vi "scan PZT_V(SubVI).vi"(0 "config":T1={"initialize"=enum."SR830", "6221"={"6221 Resource"="GPIB0::24::INSTR", "Delta status"=FALSE, "电流|RMS(A)"=0.0}, "SR830+6221"={"source"=0, "Current(A)"=0.0, "阻抗(Ohm)"=0.0, "SR830 1"=FALSE, "SR830 2"=FALSE, "SR830 3"=FALSE, "SR830 4"=FALSE, "VISA 1"="", "VISA 2"="", "VISA 3"="", "VISA 4"="", "Reserve 1"=0, "Reserve 2"=-1, "Reserve 3"=-1, "Reserve 4"=-1, "Sensitivity 1"=-1, "Sensitivity 2"=0, "Sensitivity 3"=-1, "Sensitivity 4"=-1, "量程入 1"=0, "量程入 2"=0, "量程入 3"=0, "量程入 4"=0}, "2400"={"2400"=FALSE, "VISA"="", "Output Level (0)"=1e-05, "Compliance  Level (0.1)"=10.0}, "ch"={"ch"=[], "current"=[], "change?"=[], "holding current\nwhen change ch?"=FALSE}, "Instrument"={"335 Resource"="GPIB0::24::INSTR", "Input (0:A)"=0, "Instrument Type"=enum."PPMS-Rotate", "quantum design"=refnum, "Heater Output (1:1)"=1, "semaphore"=refnum, "TCP master instance"=refnum, "335 Status"=refnum, "M24C Resource"="GPIB0::24::INSTR", "4G supply"="GPIB0::24::INSTR", "Temp Status 24C"=refnum, "Temp"=refnum, "9T信号"=refnum, "limit"={"Field limit"=0.0, "Field rate limit"=0.0, "Temp limit"=0.0, "Temp low limit"=0.0, "Temp rate limit "=0.0}, "4g supply status"=refnum, "vi路径"="", "325 Resource "="GPIB0::24::INSTR", "Input (0:A) 325"=0, "Input (1;B)"=1, "in-plane"="", "out-plane"="", "in-plane"=FALSE, "out-plane"=FALSE, "in plane 信号"=refnum, "pzt volt"=refnum, "Aborting"=refnum, "数据文件"=refnum, "warning"=refnum}, "2614B"={"2614B chA"=FALSE, "2614B chB"=FALSE, "VISA"=""}, "33522b"={"33522b resource name"="", "零电压"=0.0, "最大电压"=148.0, "间隔"=4.0, "最小电压"=-48.0, "PZT Scan?"=FALSE}, "gating type"=enum."2614(daul)"} {"Instrument"."Input (1;B)" items=["A", "B"]; "Instrument"."Input (0:A) 325" items=["A", "B"]; "Instrument"."Input (0:A)" items=["A", "B"]; "Instrument"."Heater Output (1:1)" items=["1"=1, "2"=2]; "SR830+6221"."Sensitivity 4" items=["Auto Gain"=-1, "2 nV/fA"=0, "5 nV/fA"=1, "10 nV/fA"=2, "20 nV/fA"=3, "50 nV/fA"=4, "100 nV/fA"=5, "200 nV/fA"=6, "500 nV/fA"=7, "1 uV/pA"=8, "2 uV/pA"=9, "5 uV/pA"=10, "10 uV/pA"=11, "20 uV/pA"=12, "50 uV/pA"=13, "100 uV/pA"=14, "200 uV/pA"=15, "500 uV/pA"=16, "1 mV/nA"=17, "2 mV/nA"=18, "5 mV/nA"=19, "10 mV/nA"=20, "20 mV/nA"=21, "50 mV/nA"=22, "100 mV/nA"=23, "200 mV/nA"=24, "500 mV/mA"=25, "1 V/uA"=26]; "SR830+6221"."Sensitivity 3" items=["Auto Gain"=-1, "2 nV/fA"=0, "5 nV/fA"=1, "10 nV/fA"=2, "20 nV/fA"=3, "50 nV/fA"=4, "100 nV/fA"=5, "200 nV/fA"=6, "500 nV/fA"=7, "1 uV/pA"=8, "2 uV/pA"=9, "5 uV/pA"=10, "10 uV/pA"=11, "20 uV/pA"=12, "50 uV/pA"=13, "100 uV/pA"=14, "200 uV/pA"=15, "500 uV/pA"=16, "1 mV/nA"=17, "2 mV/nA"=18, "5 mV/nA"=19, "10 mV/nA"=20, "20 mV/nA"=21, "50 mV/nA"=22, "100 mV/nA"=23, "200 mV/nA"=24, "500 mV/mA"=25, "1 V/uA"=26]; "SR830+6221"."Sensitivity 1" items=["Auto Gain"=-1, "2 nV/fA"=0, "5 nV/fA"=1, "10 nV/fA"=2, "20 nV/fA"=3, "50 nV/fA"=4, "100 nV/fA"=5, "200 nV/fA"=6, "500 nV/fA"=7, "1 uV/pA"=8, "2 uV/pA"=9, "5 uV/pA"=10, "10 uV/pA"=11, "20 uV/pA"=12, "50 uV/pA"=13, "100 uV/pA"=14, "200 uV/pA"=15, "500 uV/pA"=16, "1 mV/nA"=17, "2 mV/nA"=18, "5 mV/nA"=19, "10 mV/nA"=20, "20 mV/nA"=21, "50 mV/nA"=22, "100 mV/nA"=23, "200 mV/nA"=24, "500 mV/mA"=25, "1 V/uA"=26]; "SR830+6221"."Sensitivity 2" items=["Auto Gain"=-1, "2 nV/fA"=0, "5 nV/fA"=1, "10 nV/fA"=2, "20 nV/fA"=3, "50 nV/fA"=4, "100 nV/fA"=5, "200 nV/fA"=6, "500 nV/fA"=7, "1 uV/pA"=8, "2 uV/pA"=9, "5 uV/pA"=10, "10 uV/pA"=11, "20 uV/pA"=12, "50 uV/pA"=13, "100 uV/pA"=14, "200 uV/pA"=15, "500 uV/pA"=16, "1 mV/nA"=17, "2 mV/nA"=18, "5 mV/nA"=19, "10 mV/nA"=20, "20 mV/nA"=21, "50 mV/nA"=22, "100 mV/nA"=23, "200 mV/nA"=24, "500 mV/mA"=25, "1 V/uA"=26]; "SR830+6221"."Reserve 4" items=["Auto Gain"=-1, "2 nV/fA"=0, "5 nV/fA"=1, "10 nV/fA"=2, "20 nV/fA"=3, "50 nV/fA"=4, "100 nV/fA"=5, "200 nV/fA"=6, "500 nV/fA"=7, "1 uV/pA"=8, "2 uV/pA"=9, "5 uV/pA"=10, "10 uV/pA"=11, "20 uV/pA"=12, "50 uV/pA"=13, "100 uV/pA"=14, "200 uV/pA"=15, "500 uV/pA"=16, "1 mV/nA"=17, "2 mV/nA"=18, "5 mV/nA"=19, "10 mV/nA"=20, "20 mV/nA"=21, "50 mV/nA"=22, "100 mV/nA"=23, "200 mV/nA"=24, "500 mV/mA"=25, "1 V/uA"=26]; "SR830+6221"."Reserve 3" items=["Auto Reserve"=-1, "High Reserve"=0, "Normal"=1, "Low Noise"=2]; "SR830+6221"."Reserve 2" items=["Auto Reserve"=-1, "High Reserve"=0, "Normal"=1, "Low Noise"=2]; "SR830+6221"."Reserve 1" items=["Auto Reserve"=-1, "High Reserve"=0, "Normal"=1, "Low Noise"=2]; "SR830+6221"."source" items=["SR830 1", "SR830 2", "SR830 3", "SR830 4"]}, 12 "data":refnum<queue>) -> (4 "输出簇":T1={"initialize"=enum."SR830", "6221"={"6221 Resource"="GPIB0::24::INSTR", "Delta status"=FALSE, "电流|RMS(A)"=0.0}, "SR830+6221"={"source"=0, "Current(A)"=0.0, "阻抗(Ohm)"=0.0, "SR830 1"=FALSE, "SR830 2"=FALSE, "SR830 3"=FALSE, "SR830 4"=FALSE, "VISA 1"="", "VISA 2"="", "VISA 3"="", "VISA 4"="", "Reserve 1"=0, "Reserve 2"=-1, "Reserve 3"=-1, "Reserve 4"=-1, "Sensitivity 1"=-1, "Sensitivity 2"=0, "Sensitivity 3"=-1, "Sensitivity 4"=-1, "量程入 1"=0, "量程入 2"=0, "量程入 3"=0, "量程入 4"=0}, "2400"={"2400"=FALSE, "VISA"="", "Output Level (0)"=1e-05, "Compliance  Level (0.1)"=10.0}, "ch"={"ch"=[], "current"=[], "change?"=[], "holding current\nwhen change ch?"=FALSE}, "Instrument"={"335 Resource"="GPIB0::24::INSTR", "Input (0:A)"=0, "Instrument Type"=enum."PPMS-Rotate", "quantum design"=refnum, "Heater Output (1:1)"=1, "semaphore"=refnum, "TCP master instance"=refnum, "335 Status"=refnum, "M24C Resource"="GPIB0::24::INSTR", "4G supply"="GPIB0::24::INSTR", "Temp Status 24C"=refnum, "Temp"=refnum, "9T信号"=refnum, "limit"={"Field limit"=0.0, "Field rate limit"=0.0, "Temp limit"=0.0, "Temp low limit"=0.0, "Temp rate limit "=0.0}, "4g supply status"=refnum, "vi路径"="", "325 Resource "="GPIB0::24::INSTR", "Input (0:A) 325"=0, "Input (1;B)"=1, "in-plane"="", "out-plane"="", "in-plane"=FALSE, "out-plane"=FALSE, "in plane 信号"=refnum, "pzt volt"=refnum, "Aborting"=refnum, "数据文件"=refnum, "warning"=refnum}, "2614B"={"2614B chA"=FALSE, "2614B chB"=FALSE, "VISA"=""}, "33522b"={"33522b resource name"="", "零电压"=0.0, "最大电压"=148.0, "间隔"=4.0, "最小电压"=-48.0, "PZT Scan?"=FALSE}, "gating type"=enum."2614(daul)"} {"Instrument"."Input (1;B)" items=["A", "B"]; "Instrument"."Input (0:A) 325" items=["A", "B"]; "Instrument"."Input (0:A)" items=["A", "B"]; "Instrument"."Heater Output (1:1)" items=["1"=1, "2"=2]; "SR830+6221"."Sensitivity 4" items=["Auto Gain"=-1, "2 nV/fA"=0, "5 nV/fA"=1, "10 nV/fA"=2, "20 nV/fA"=3, "50 nV/fA"=4, "100 nV/fA"=5, "200 nV/fA"=6, "500 nV/fA"=7, "1 uV/pA"=8, "2 uV/pA"=9, "5 uV/pA"=10, "10 uV/pA"=11, "20 uV/pA"=12, "50 uV/pA"=13, "100 uV/pA"=14, "200 uV/pA"=15, "500 uV/pA"=16, "1 mV/nA"=17, "2 mV/nA"=18, "5 mV/nA"=19, "10 mV/nA"=20, "20 mV/nA"=21, "50 mV/nA"=22, "100 mV/nA"=23, "200 mV/nA"=24, "500 mV/mA"=25, "1 V/uA"=26]; "SR830+6221"."Sensitivity 3" items=["Auto Gain"=-1, "2 nV/fA"=0, "5 nV/fA"=1, "10 nV/fA"=2, "20 nV/fA"=3, "50 nV/fA"=4, "100 nV/fA"=5, "200 nV/fA"=6, "500 nV/fA"=7, "1 uV/pA"=8, "2 uV/pA"=9, "5 uV/pA"=10, "10 uV/pA"=11, "20 uV/pA"=12, "50 uV/pA"=13, "100 uV/pA"=14, "200 uV/pA"=15, "500 uV/pA"=16, "1 mV/nA"=17, "2 mV/nA"=18, "5 mV/nA"=19, "10 mV/nA"=20, "20 mV/nA"=21, "50 mV/nA"=22, "100 mV/nA"=23, "200 mV/nA"=24, "500 mV/mA"=25, "1 V/uA"=26]; "SR830+6221"."Sensitivity 1" items=["Auto Gain"=-1, "2 nV/fA"=0, "5 nV/fA"=1, "10 nV/fA"=2, "20 nV/fA"=3, "50 nV/fA"=4, "100 nV/fA"=5, "200 nV/fA"=6, "500 nV/fA"=7, "1 uV/pA"=8, "2 uV/pA"=9, "5 uV/pA"=10, "10 uV/pA"=11, "20 uV/pA"=12, "50 uV/pA"=13, "100 uV/pA"=14, "200 uV/pA"=15, "500 uV/pA"=16, "1 mV/nA"=17, "2 mV/nA"=18, "5 mV/nA"=19, "10 mV/nA"=20, "20 mV/nA"=21, "50 mV/nA"=22, "100 mV/nA"=23, "200 mV/nA"=24, "500 mV/mA"=25, "1 V/uA"=26]; "SR830+6221"."Sensitivity 2" items=["Auto Gain"=-1, "2 nV/fA"=0, "5 nV/fA"=1, "10 nV/fA"=2, "20 nV/fA"=3, "50 nV/fA"=4, "100 nV/fA"=5, "200 nV/fA"=6, "500 nV/fA"=7, "1 uV/pA"=8, "2 uV/pA"=9, "5 uV/pA"=10, "10 uV/pA"=11, "20 uV/pA"=12, "50 uV/pA"=13, "100 uV/pA"=14, "200 uV/pA"=15, "500 uV/pA"=16, "1 mV/nA"=17, "2 mV/nA"=18, "5 mV/nA"=19, "10 mV/nA"=20, "20 mV/nA"=21, "50 mV/nA"=22, "100 mV/nA"=23, "200 mV/nA"=24, "500 mV/mA"=25, "1 V/uA"=26]; "SR830+6221"."Reserve 4" items=["Auto Gain"=-1, "2 nV/fA"=0, "5 nV/fA"=1, "10 nV/fA"=2, "20 nV/fA"=3, "50 nV/fA"=4, "100 nV/fA"=5, "200 nV/fA"=6, "500 nV/fA"=7, "1 uV/pA"=8, "2 uV/pA"=9, "5 uV/pA"=10, "10 uV/pA"=11, "20 uV/pA"=12, "50 uV/pA"=13, "100 uV/pA"=14, "200 uV/pA"=15, "500 uV/pA"=16, "1 mV/nA"=17, "2 mV/nA"=18, "5 mV/nA"=19, "10 mV/nA"=20, "20 mV/nA"=21, "50 mV/nA"=22, "100 mV/nA"=23, "200 mV/nA"=24, "500 mV/mA"=25, "1 V/uA"=26]; "SR830+6221"."Reserve 3" items=["Auto Reserve"=-1, "High Reserve"=0, "Normal"=1, "Low Noise"=2]; "SR830+6221"."Reserve 2" items=["Auto Reserve"=-1, "High Reserve"=0, "Normal"=1, "Low Noise"=2]; "SR830+6221"."Reserve 1" items=["Auto Reserve"=-1, "High Reserve"=0, "Normal"=1, "Low Noise"=2]; "SR830+6221"."source" items=["SR830 1", "SR830 2", "SR830 3", "SR830 4"]}, 6 "错误输出":errorcluster)   [LabVIEW 2019, in "nematic.lvlib"]
uses:
  nematic.lvlib
  ctl/config.ctl
  <vilib>/NI/Modbus Library/API/Master/Modbus Master.lvclass
  ctl/initialize.ctl
  ctl/Instrument.ctl
  ctl/Instrument Type.ctl
  lib/QDInstrument.dll
  ctl/335 state.ctl
  ctl/limit.ctl
  ctl/9T mag field stauts.ctl
  ctl/warning.ctl
  ctl/Gating type.ctl
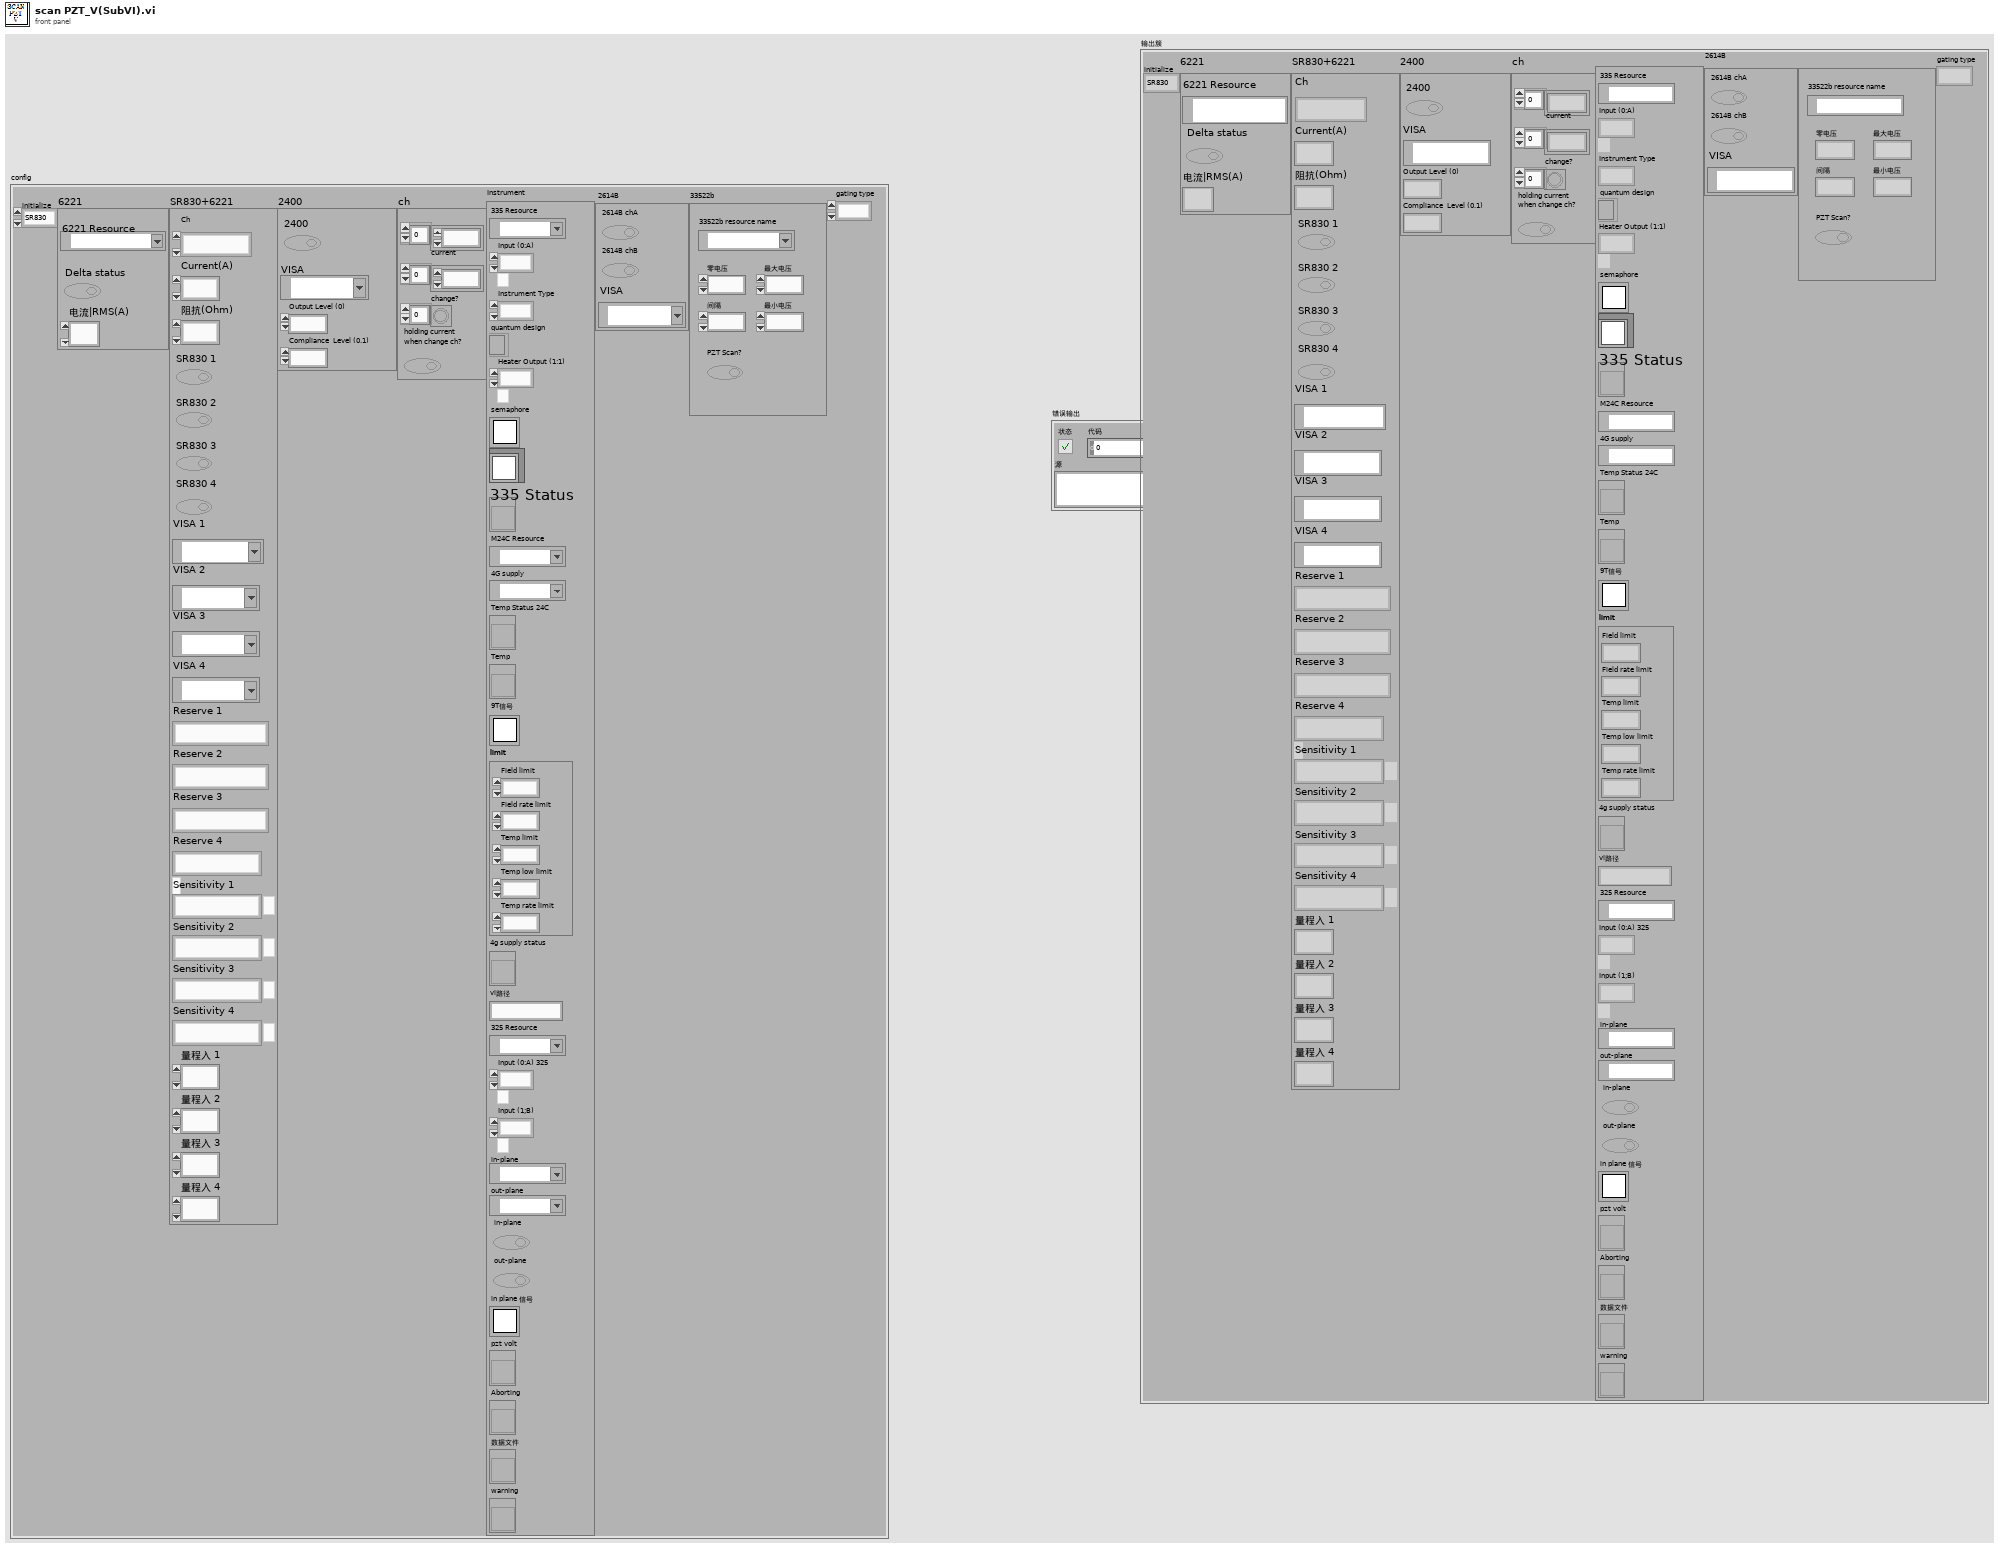
[diagram p1: front panel]
types:
  T1 = typedef "config.ctl" = cluster{"initialize":T2, "6221":cluster{"6221 Resource":refnum<visa-resource-name>, "Delta status":bool, "电流|RMS(A)":dbl}, "SR830+6221":cluster{"source":u16, "Current(A)":dbl, "阻抗(Ohm)":dbl, "SR830 1":bool, "SR830 2":bool, "SR830 3":bool, "SR830 4":bool, "VISA 1":refnum<visa-resource-name>, "VISA 2":refnum<visa-resource-name>, "VISA 3":refnum<visa-resource-name>, "VISA 4":refnum<visa-resource-name>, "Reserve 1":i16, "Reserve 2":i16, "Reserve 3":i16, "Reserve 4":i16, "Sensitivity 1":i16, "Sensitivity 2":i16, "Sensitivity 3":i16, "Sensitivity 4":i16, "量程入 1":i32, "量程入 2":i32, "量程入 3":i32, "量程入 4":i32}, "2400":cluster{"2400":bool, "VISA":refnum<visa-resource-name>, "Output Level (0)":dbl, "Compliance  Level (0.1)":dbl}, "ch":cluster{"ch":i32[], "current":dbl[], "change?":bool[], "holding current\nwhen change ch?":bool}, "Instrument":T3, "2614B":cluster{"2614B chA":bool, "2614B chB":bool, "VISA":refnum<visa-resource-name>}, "33522b":cluster{"33522b resource name":refnum<visa-resource-name>, "零电压":dbl, "最大电压":dbl, "间隔":dbl, "最小电压":dbl, "PZT Scan?":bool}, "gating type":T7}
  T2 = typedef "initialize.ctl" = enum16{"SR830", "keithley6221-SR830", "Delta", "Delta-tunnelling", "keithley6221-2182-DC", "PZT"}
  T3 = typedef "Instrument.ctl" = cluster{"335 Resource":refnum<visa-resource-name>, "Input (0:A)":u16, "Instrument Type":T4, "quantum design":refnum<k24>, "Heater Output (1:1)":u16, "semaphore":T5, "TCP master instance":refnum<class "Modbus Master.lvclass">, "335 Status":refnum<vi>, "M24C Resource":refnum<visa-resource-name>, "4G supply":refnum<visa-resource-name>, "Temp Status 24C":refnum<vi>, "Temp":refnum<vi>, "9T信号":T5, "limit":T6, "4g supply status":refnum<vi>, "vi路径":string, "325 Resource ":refnum<visa-resource-name>, "Input (0:A) 325":u16, "Input (1;B)":u16, "in-plane":refnum<visa-resource-name>, "out-plane":refnum<visa-resource-name>, "in-plane":bool, "out-plane":bool, "in plane 信号":T5, "pzt volt":refnum<vi>, "Aborting":refnum<vi>, "数据文件":refnum<vi>, "warning":refnum<vi>}
  T4 = typedef "Instrument Type.ctl" = enum16{"PPMS", "VersaLab", "DynaCool", "SVSM", "PPMS-Rotate", "Lakeshore335", "lengtou2", "9T mag", "9T cmag rotate", "test"}
  T5 = typedef "Semaphore RefNum" = refnum<k1>
  T6 = typedef "limit.ctl" = cluster{"Field limit":dbl, "Field rate limit":dbl, "Temp limit":dbl, "Temp low limit":dbl, "Temp rate limit ":dbl}
  T7 = typedef "Gating type.ctl" = enum32{"null", "2614(daul)", "2400"}
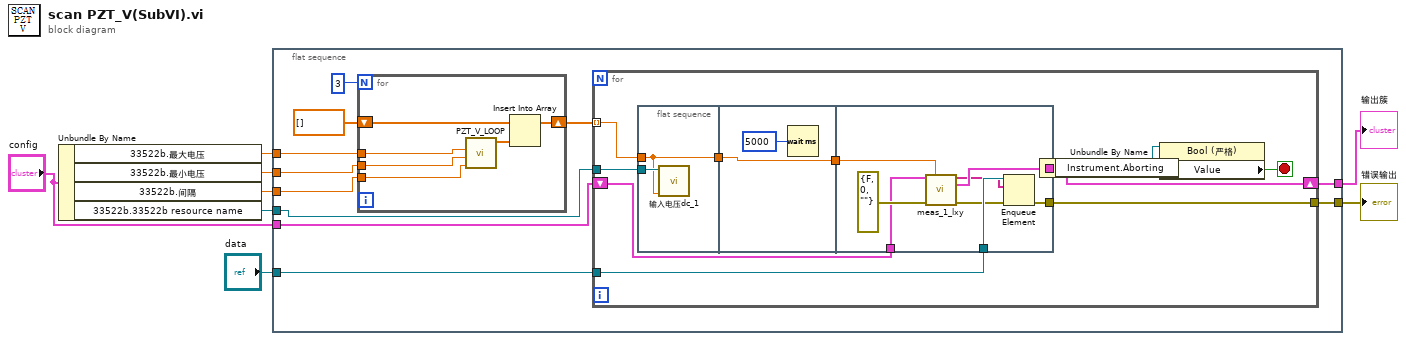
[diagram p0: block diagram]
diagram:
  n1 = Unbundle By Name("config") -> ("33522b.最大电压"=w3:dbl, "33522b.最小电压"=w2:dbl, "33522b.间隔"=w1:dbl, "33522b.33522b resource name"=w4:refnum<visa-resource-name>)
  n2 = flat-sequence {
    tunnel: w4 -> [w18]
    tunnel: [w14] -> w7
    tunnel: "config" -> [w15]
    tunnel: "data" -> [w16]
    tunnel: [w13] -> w6
    tunnel: w3 -> [w11]
    tunnel: w1 -> [w10]
    tunnel: w2 -> [w9]
    frame #0 {
      n3 = for {
        N: 3 -> [_]
        shift-right: [w47] -> w19
        shift-left: dbl[] [] -> [w46]
        tunnel: w11 -> [w45]
        tunnel: w9 -> [w44]
        tunnel: w10 -> [w43]
        n4 = call "PZT_V_LOOP.vi"("间隔"=w43, "最小电压"=w44, "最大电压"=w45) -> ("output array"=w42:dbl[])  [unwired: 8 in]
        n5 = Insert Into Array(array=w46, new element=w42) -> (w47:dbl[])  [unwired: 1 in]
      }
      n6 = for {
        tunnel: w19 -> [w28] mode=indexing
        tunnel: w18 -> [w29]
        tunnel: w16 -> [w27]
        tunnel: [w25] -> w14
        shift-right: [w22] -> w13
        shift-left: w15 -> [w26]
        stop <- w23 stop-if-true
        n7 = flat-sequence {
          tunnel: w29 -> [w31]
          tunnel: w28 -> [w30]
          tunnel: [w30] -> w21
          tunnel: w21 -> [w32]
          tunnel: [w32] -> w20
          tunnel: w27 -> [w41]
          tunnel: w26 -> [w39]
          tunnel: [w38] -> w22
          tunnel: [w37] -> w25
          tunnel: w20 -> [w36]
          frame #0 {
            n8 = call "输入电压dc_1.vi"("压电陶瓷电压 (0.1 Vpp)"=w30, "33522b resource name"=w31) -> ()  [unwired: 5 in]
          }
          frame #1 {
            n9 = Wait (ms)(milliseconds to wait=u32 5000 ("等待时间（毫秒）")) -> ()  [unwired: 1 out]
          }
          frame #2 {
            n10 = call "meas_1_lxy.vi"("config"=w39, "压电陶瓷电压 (Vpp)"=w36, "错误输入（无错误）"=errorcluster {"status"=FALSE, "code"=0, "source"=""} ("error out")) -> ("数组"=w34:string[], "输出簇"=w38:T1, "错误输出"=w35:errorcluster)  [unwired: 10 in]
            n11 = Enqueue Element(queue=w41, element=w34, error in (no error)=w35) -> (error out=w37:errorcluster)  [unwired: 1 in, 2 out]
          }
        }
        n12 = Unbundle By Name(w22) -> ("Instrument.Aborting"=w24:refnum<vi>)
        n13 = property class="Bool (严格)"(reference=w24) -> ("Value"=w23:bool)  [unwired: 1 in, 2 out]
      }
    }
  }
  "错误输出" <- w7
  "输出簇" <- w6
